vi "GuardaValorsPantalla.vi"(0 "Rings":refnum<vi>[](array[refnum]), 1 "Caselles":refnum<vi>[](array[refnum]), 2 "Booleans":refnum<vi>[](array[refnum])) -> (10 "error out":errorcluster)   [LabVIEW 2017]
uses:
  <vilib>/registry/registry.llb/Registry RtKey.ctl
  <vilib>/registry/registry.llb/Write Registry Value Simple STR.vi
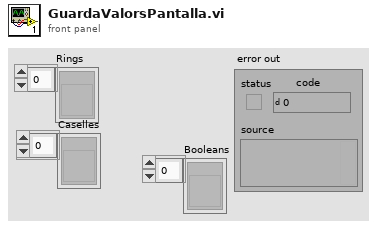
[diagram p1: front panel]
types:
  T1 = typedef "Registry RtKey.ctl" = enum32{"HKEY_CLASSES_ROOT", "HKEY_CURRENT_USER", "HKEY_LOCAL_MACHINE", "HKEY_USERS", "HKEY_PERFORMANCE_DATA", "HKEY_CURRENT_CONFIG", "HKEY_DYN_DATA"}
  T2 = typedef "Registry refnum.ctl" = refnum<k1>
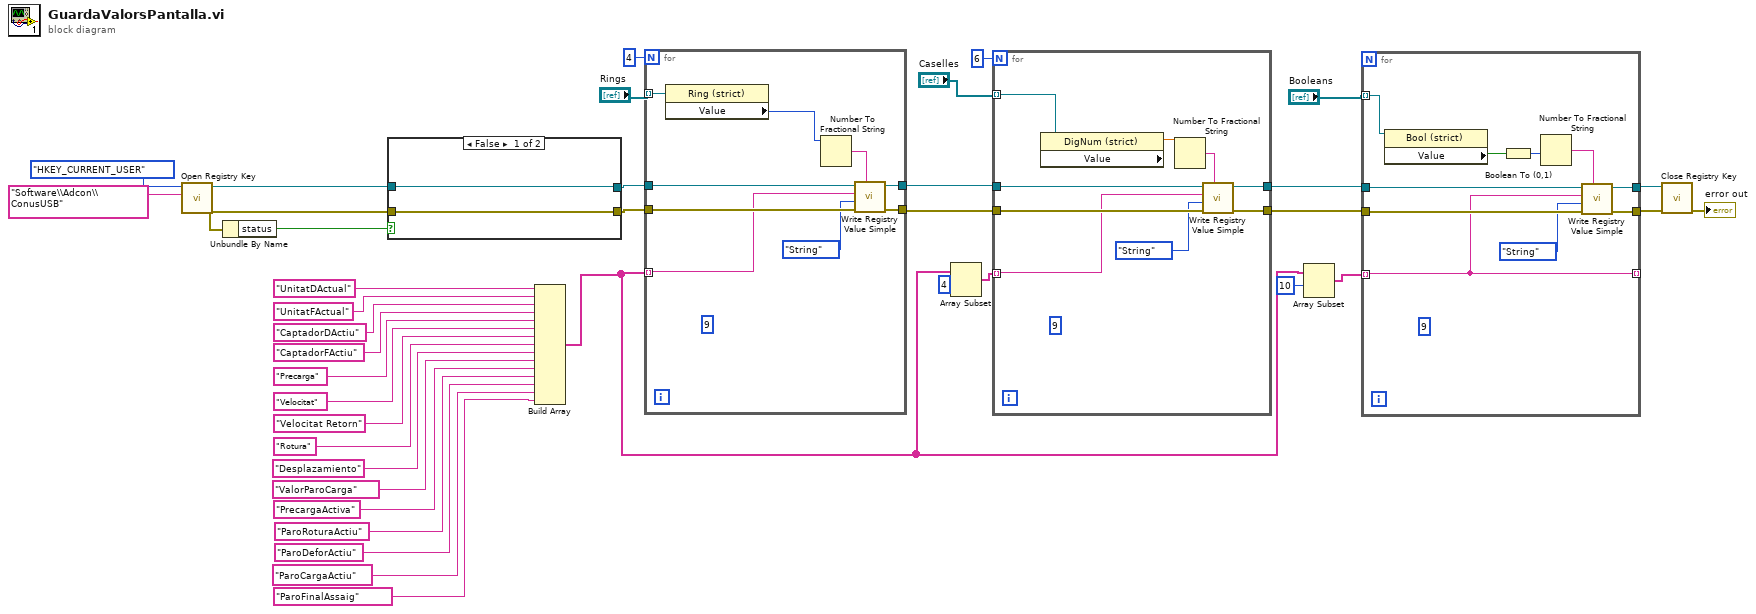
[diagram p0: block diagram]
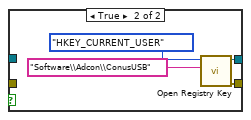
[diagram p2: hidden frame]
diagram:
  n1 = call <vilib>:"Open Registry Key.vi"("subkey"="Software\\Adcon\\ConusUSB", "root key (HKEY_LOCAL_MACHINE)"=Registry_RtKey."HKEY_CURRENT_USER") -> ("error out"=w2:errorcluster, "refnum out"=w3:T2)  [unwired: 8 in]
  n2 = Unbundle By Name(w2) -> ("status"=w4:bool)
  n3 = case shown="False" w4 {
    tunnel: [w41 w43] -> w39
    tunnel: [w40 w42] -> w38
    tunnel: w3 -> [w41 _]
    tunnel: w2 -> [w40 _]
    frame False {
    }
    frame True {
      n4 = call <vilib>:"Open Registry Key.vi"("subkey"="Software\\Adcon\\ConusUSB", "root key (HKEY_LOCAL_MACHINE)"=Registry_RtKey."HKEY_CURRENT_USER") -> ("error out"=w42:errorcluster, "refnum out"=w43:T2)  [unwired: 8 in]
    }
  }
  n5 = Build Array("UnitatDActual" ("value"), "UnitatFActual" ("value"), "CaptadorDActiu" ("value"), "CaptadorFActiu" ("value"), "Precarga" ("value"), "Velocitat" ("value"), "Velocitat Retorn" ("value"), "Rotura" ("value"), "Desplazamiento" ("value"), "ValorParoCarga" ("value"), "PrecargaActiva" ("value"), "ParoRoturaActiu" ("value"), "ParoDeforActiu" ("value"), "ParoCargaActiu" ("value"), "ParoFinalAssaig" ("value")) -> (w24:string[])
  n6 = for {
    N: 4 -> [_]
    tunnel: "Rings" -> [w54] mode=indexing
    tunnel: w39 -> [w53]
    tunnel: w24 -> [w47] mode=indexing
    tunnel: w38 -> [w52]
    tunnel: [w51] -> w35
    tunnel: [w50] -> w34
    (unwired) 9 ("y")
    n7 = property class="Ring (strict)"(reference=w54) -> ("Value"=w46:u16)  [unwired: 1 in, 2 out]
    n8 = Number To Fractional String(number=w46) -> (F-format string=w49:string)  [unwired: 3 in]
    n9 = call-poly <vilib>:"Write Registry Value Simple.vi"("String/Binary data"=w49, "error in (no error)"=w52, "simple data type"=enum16{"String", "Binary", "DWORD"}."String", "value"=w47, "refnum"=w53) -> ("error out"=w50:errorcluster, "refnum out"=w51:T2)  [unwired: 3 in]
  }
  n10 = Array Subset(array=w24, index=4) -> (w33:string[])  [unwired: 1 in]
  n11 = for {
    N: 6 -> [_]
    tunnel: "Caselles" -> [w63] mode=indexing
    tunnel: w35 -> [w62]
    tunnel: w33 -> [w56] mode=indexing
    tunnel: w34 -> [w61]
    tunnel: [w60] -> w30
    tunnel: [w59] -> w29
    (unwired) 9 ("y")
    n12 = property class="DigNum (strict)"(reference=w63) -> ("Value"=w55:sgl)  [unwired: 1 in, 2 out]
    n13 = Number To Fractional String(number=w55) -> (F-format string=w58:string)  [unwired: 3 in]
    n14 = call-poly <vilib>:"Write Registry Value Simple.vi"("String/Binary data"=w58, "error in (no error)"=w61, "simple data type"=enum16{"String", "Binary", "DWORD"}."String", "value"=w56, "refnum"=w62) -> ("error out"=w59:errorcluster, "refnum out"=w60:T2)  [unwired: 3 in]
  }
  n15 = Array Subset(array=w24, index=10) -> (w27:string[])  [unwired: 1 in]
  n16 = for {
    tunnel: "Booleans" -> [w66] mode=indexing
    tunnel: w30 -> [w73]
    tunnel: w27 -> [w67] mode=indexing
    tunnel: w29 -> [w72]
    tunnel: [w71] -> w26
    tunnel: [w70] -> w25
    tunnel: [w67] -> _ mode=indexing
    (unwired) 9 ("y")
    n17 = property class="Bool (strict)"(reference=w66) -> ("Value"=w64:bool)  [unwired: 1 in, 2 out]
    n18 = Boolean To (0,1)(Boolean=w64) -> (0, 1=w65:i16)
    n19 = Number To Fractional String(number=w65) -> (F-format string=w69:string)  [unwired: 3 in]
    n20 = call-poly <vilib>:"Write Registry Value Simple.vi"("String/Binary data"=w69, "error in (no error)"=w72, "simple data type"=enum16{"String", "Binary", "DWORD"}."String", "value"=w67, "refnum"=w73) -> ("error out"=w70:errorcluster, "refnum out"=w71:T2)  [unwired: 3 in]
  }
  n21 = call <vilib>:"Close Registry Key.vi"("error in (no error)"=w25, "refnum"=w26) -> ("error out"=→"error out":errorcluster)  [unwired: 5 in]
